vi "generate output command.vi"(6 "messageHandler":T1 {"params"."controlChannels"."ballControl" items=["Module6/output0", "Module6/output1", "Module6/output2", "Module6/output3", "Not-Used"]; "params"."controlChannels"."butterflyControl" items=["Module6/output0", "Module6/output1", "Module6/output2", "Module6/output3", "Not-Used"]; "params"."controlChannels"."speedControl" items=["Module6/output0", "Module6/output1", "Module6/output2", "Module6/output3", "Not-Used"]}, 9 "control data":variant, 11 "Queues in":T2) -> ()   [LabVIEW 2018]
uses:
  type defs/Queues.ctl
  type defs/message handler data.ctl
  customVI/liveData/state.ctl
  supporting VIs/polymorphic VIs/enqueue for file IO.vi
  supporting VIs/polymorphic VIs/enqueue for custom.vi
  RT/Message Handler loop/FPGA commands/RT - FPGA commands.lvlib
panel:
  out "command type":string
  out "channel index":u16
  out "voltage":dbl
  out "command value":dbl
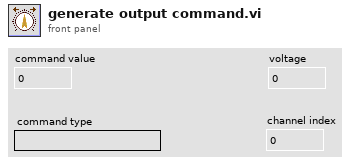
[diagram p1: front panel]
types:
  T1 = typedef "message handler data.ctl" = cluster{"params":cluster{"configFileID":u32, "configFilePath":path, "channelConfigFilePath":path, "incidentLogfile":path, "controlChannels":cluster{"ballControl":u16, "butterflyControl":u16, "speedControl":u16}, "pulsatorVIPath":path, "customVIPath":path, "HowdenAir":cluster{"vent Howden":bool, "Howden%":dbl}}, "vars":cluster{"commsStatus":bool[], "controlIndex":cluster{"ballControl":u16, "butterflyControl":u16, "speedControl":u16}, "customVIRef":refnum<vi>, "Interlocks":cluster{"gearboxOil":bool, "bearingOil":bool, "gearboxAir":bool}, "motorRunning":bool, "liveDataQ":refnum<queue>[]}}
  T2 = typedef "Queues.ctl" = cluster{"messageHandler":refnum<queue>, "comms":refnum<queue>, "dataStream":refnum<queue>, "dataProcessor":refnum<queue>, "fileIO":refnum<queue>, "userInterface":refnum<queue>, "errors":refnum<queue>, "customCompressor":refnum<queue>}
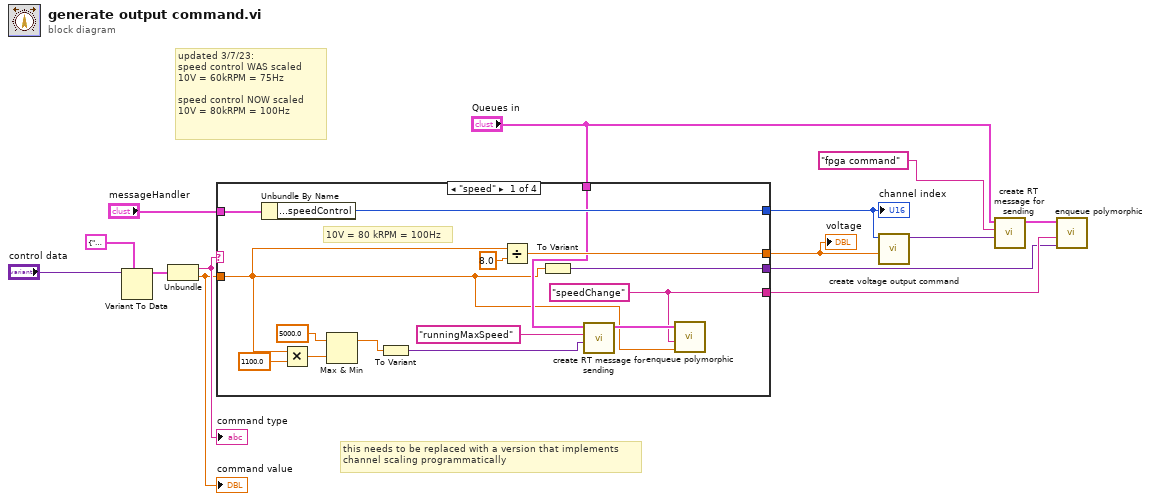
[diagram p0: block diagram]
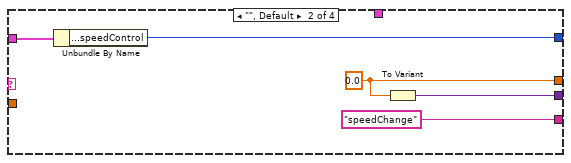
[diagram p2: hidden frame]
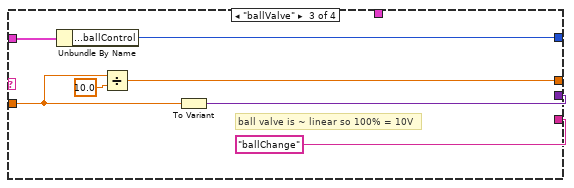
[diagram p3: hidden frame]
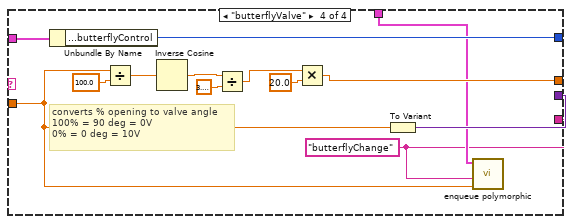
[diagram p4: hidden frame]
diagram:
  # "updated 3/7/23:\nspeed control WAS scaled \n10V = 60kRPM = 75Hz\n\nspeed control NOW scaled\n10V = 80kRPM = 100Hz"
  # "this needs to be replaced with a version that implements\nchannel scaling programmatically"
  n1 = Variant To Data(type=cluster{string, dbl} {"", 0.0}, Variant="control data") -> (data=w12:cluster{string, dbl})  [unwired: 1 in, 1 out]
  n2 = Unbundle(w12) -> (w13:string, w8:dbl)
  "command value" <- w8
  "command type" <- w13
  n3 = case shown="\"speed\"" w13 {
    tunnel: "messageHandler" -> [w29 w34 w41 w54]
    tunnel: [w28 w33 w40 w53] -> w9
    tunnel: [w27 w31 w39 w45] -> w7
    tunnel: w8 -> [w15 _ w35 w42]
    tunnel: [w16 "speedChange" ("message") "ballChange" ("message") w43] -> w3
    tunnel: [w25 w30 w36 w49] -> w2
    tunnel: "Queues in" -> [w24 _ _ w44]
    frame "speed" {
      w16 = "speedChange" ("message")
      # "10V = 80 kRPM = 100Hz"
      n4 = Unbundle By Name(w29) -> ("vars.controlIndex.speedControl"=w28:u16)
      n5 = Multiply(x=w15, y=1100.0) -> (x*y=w21:dbl)
      n6 = Max & Min(x=5000.0 ("y"), y=w21) -> (max(x,y)=w19:dbl)  [unwired: 1 out]
      n7 = To Variant(anything=w19) -> (Variant=w18:variant)
      n8 = Divide(x=w15, y=8.0) -> (x/y=w27:dbl)
      n9 = To Variant(anything=w15) -> (Variant=w25:variant)
      n10 = call "create RT message for sending.vi"("RT data"=w18, "RT message"="runningMaxSpeed", "Queues in"=w24) -> ("Queues out"=w17:T2)  [unwired: 8 in]
      n11 = call-poly "enqueue polymorphic.vi"("data"=w15, "message"=w16, "Queues"=w17) -> ()  [unwired: 8 in, 1 out]
    }
    frame "", Default {
      w31 = 0.0
      n12 = Unbundle By Name(w34) -> ("vars.controlIndex.speedControl"=w33:u16)
      n13 = To Variant(anything=w31) -> (Variant=w30:variant)
    }
    frame "ballValve" {
      # "ball valve is ~ linear so 100% = 10V"
      n14 = Unbundle By Name(w41) -> ("vars.controlIndex.ballControl"=w40:u16)
      n15 = Divide(x=w35, y=10.0) -> (x/y=w39:dbl)
      n16 = To Variant(anything=w35) -> (Variant=w36:variant)
    }
    frame "butterflyValve" {
      w43 = "butterflyChange" ("message")
      # "converts % opening to valve angle\n100% = 90 deg = 0V\n0% = 0 deg = 10V"
      n17 = Unbundle By Name(w54) -> ("vars.controlIndex.butterflyControl"=w53:u16)
      n18 = Divide(x=w42, y=100.0) -> (x/y=w48:dbl)
      n19 = Inverse Cosine(1:w48) -> (0:w47:dbl)
      n20 = Divide(x=w47, y=3.141592653589793) -> (x/y=w46:dbl)
      n21 = Multiply(x=w46, y=20.0) -> (x*y=w45:dbl)
      n22 = To Variant(anything=w42) -> (Variant=w49:variant)
      n23 = call-poly "enqueue polymorphic.vi"("data"=w42, "message"=w43, "Queues"=w44) -> ()  [unwired: 8 in, 1 out]
    }
  }
  "voltage" <- w7
  "channel index" <- w9
  n24 = call "create voltage output command.vi"("new output (V)"=w7, "channel"=w9) -> ("command message"=w6:variant)  [unwired: 9 in]
  n25 = call "create RT message for sending.vi"("RT data"=w6, "RT message"="fpga command", "Queues in"="Queues in") -> ("Queues out"=w4:T2)  [unwired: 8 in]
  n26 = call-poly "enqueue polymorphic.vi"("data"=w2, "message"=w3, "Queues"=w4) -> ()  [unwired: 8 in, 1 out]
